vi "Chapter2Part2.vi"() -> ()   [LabVIEW 2014]
panel:
  out "Array 2":dbl[](array[numeric])
  out "Array":dbl[](array[numeric])
  out "Waveform Graph":cluster{dbl, dbl, dbl[]}(graph)
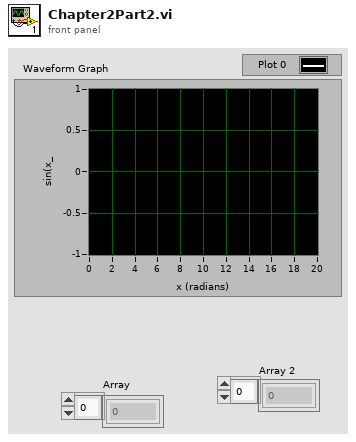
[diagram p1: front panel]
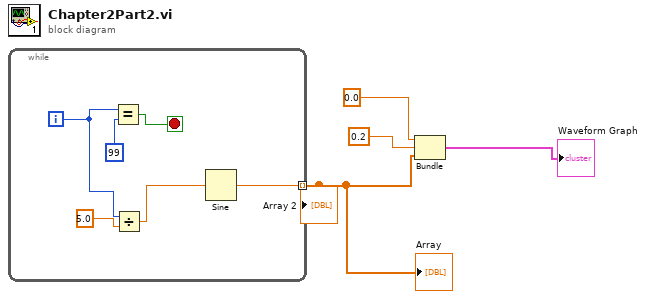
[diagram p0: block diagram]
diagram:
  n1 = while {
    tunnel: [w5] -> w1 mode=indexing
    i -> [w8]
    stop <- w7 stop-if-true
    n2 = Equal?(x=w8, y=99) -> (x = y?=w7:bool)
    n3 = Divide(x=w8, y=5.0) -> (x/y=w6:dbl)
    n4 = Sine(x=w6) -> (sin(x)=w5:dbl)
  }
  "Array" <- w1
  "Array 2" <- w1
  n5 = Bundle(0.0, 0.2, w1) -> (→"Waveform Graph":cluster{dbl, dbl, dbl[]})  [unwired: 1 in]
